vi "SetAngleDecel.vi"(1 "tf":dbl, 2 "w":dbl, 3 "tc":dbl, 4 "ta":dbl, 5 "t":dbl, 6 "a":dbl) -> (0 "CurrentAngle":dbl)   [LabVIEW 2015]
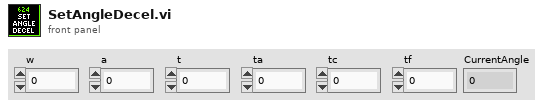
[diagram p1: front panel]
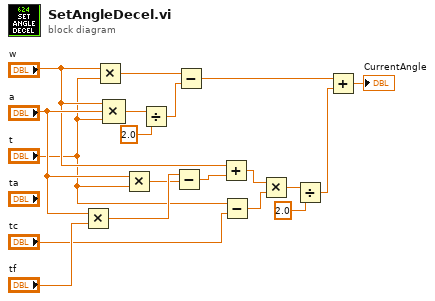
[diagram p0: block diagram]
diagram:
  n1 = Multiply(x="a", y="tf") -> (x*y=w16:dbl)
  n2 = Multiply(x="w", y="t") -> (x*y=w19:dbl)
  n3 = Compound Arithmetic op=MULTIPLY("w", "a", "t") -> (w5:dbl)
  n4 = Multiply(x="a", y="t") -> (x*y=w15:dbl)
  n5 = Divide(x=w5, y=2.0) -> (x/y=w4:dbl)
  n6 = Subtract(x=w16, y=w15) -> (x-y=w13:dbl)
  n7 = Subtract(x=w19, y=w4) -> (x-y=w3:dbl)
  n8 = Add(x="w", y=w13) -> (x+y=w10:dbl)
  n9 = Subtract(x="t", y="tc") -> (x-y=w9:dbl)
  n10 = Multiply(x=w10, y=w9) -> (x*y=w7:dbl)
  n11 = Divide(x=w7, y=2.0) -> (x/y=w2:dbl)
  n12 = Add(x=w3, y=w2) -> (x+y=→"CurrentAngle":dbl)
